vi "lifetimeparameters.vi"(1 "Params in":T1={"initialized"=FALSE, "devidx"=0, "Ch0 Level"=0, "Ch0 ZeroX"=0, "Ch1 Level"=0, "Ch1 ZeroX"=0, "sync rate"=0, "resolution"=0, "acq time"=0, "acq rate"=0, "# bins"=0, "Bin size"=enum."1", "min photons"=1, "truncate"=0} {"acq rate" step=512; "truncate" min=1; "min photons" min=1}, 2 "command":string="clear") -> (0 "Params out":T1={"initialized"=FALSE, "devidx"=0, "Ch0 Level"=70, "Ch0 ZeroX"=10, "Ch1 Level"=300, "Ch1 ZeroX"=10, "sync rate"=80000000, "resolution"=4, "acq time"=1000, "acq rate"=131072, "# bins"=13, "Bin size"=enum."1", "min photons"=5, "truncate"=3})   [LabVIEW 2015]
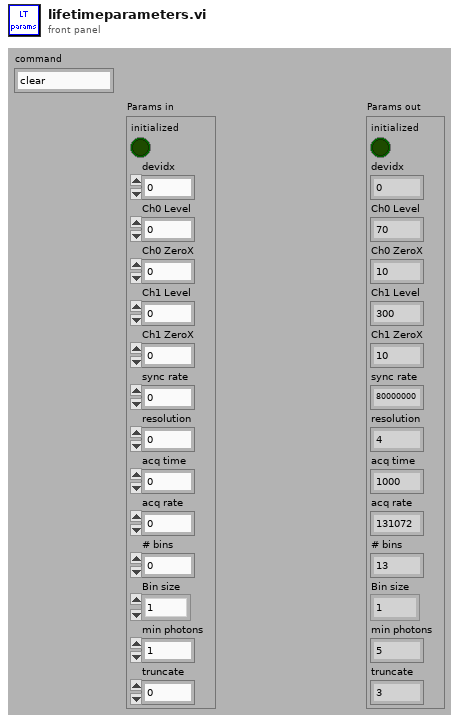
[diagram p1: front panel]
types:
  T1 = cluster{"initialized":bool, "devidx":i32, "Ch0 Level":i32, "Ch0 ZeroX":i32, "Ch1 Level":i32, "Ch1 ZeroX":i32, "sync rate":i32, "resolution":i32, "acq time":i32, "acq rate":i32, "# bins":u32, "Bin size":enum16{"1", "2", "4", "8", "16", "32", "64", "128"}, "min photons":u32, "truncate":u32}
  T2 = enum16{"1", "2", "4", "8", "16", "32", "64", "128"}
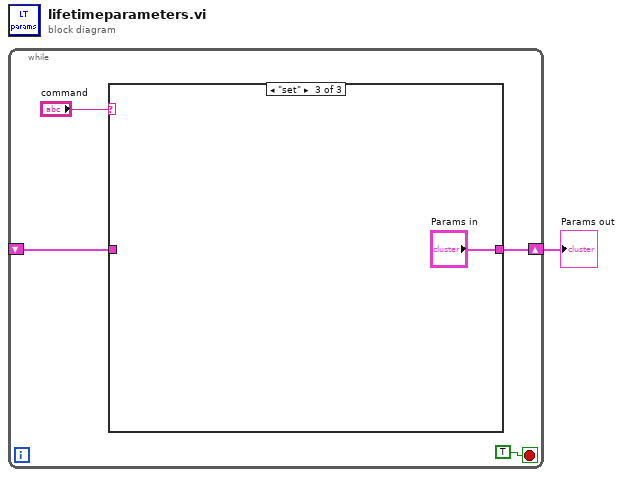
[diagram p0: block diagram]
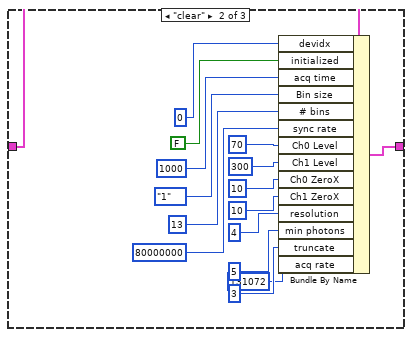
[diagram p3: hidden frame]
diagram:
  n1 = while {
    shift-right: [w3] -> w1
    shift-left: _ -> [w2]
    stop <- TRUE stop-if-true
    n2 = case shown="\"set\"" "command" {
      tunnel: [w6 w21 "Params in"] -> w3
      tunnel: w2 -> [w6 w22 _]
      frame "get", Default {
      }
      frame "clear" {
        n3 = Bundle By Name(cluster=w22, "devidx"=0, "initialized"=FALSE, "acq time"=1000, "Bin size"=T2."1", "# bins"=u32 13, "sync rate"=80000000, "Ch0 Level"=70, "Ch1 Level"=300, "Ch0 ZeroX"=10, "Ch1 ZeroX"=10, "resolution"=4, "min photons"=u32 5, "truncate"=u32 3, "acq rate"=131072) -> (w21:T1)
      }
      frame "set" {
      }
    }
  }
  "Params out" <- w1
